vi "Passing Paramters Complex Struct.vi"(7 "y":i32, 9 "x":i32, 10 "numVertices":i32, 11 "name":u32) -> (3 "function return":i32)   [LabVIEW 2018, in "ParsingDataSampleDLL.lvlib"]
doc: "__declspec(dllexport) int PassingParamters_ComplexStruct (struct complexStructPolygon triangle);"
uses:
  ParsingDataSampleDLL.lvlib
  ni_reference_vs/Debug/ParsingDataSampleDLL.dll
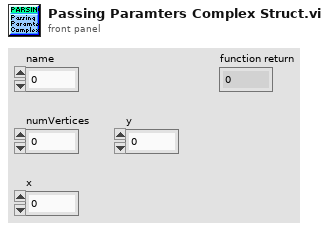
[diagram p1: front panel]
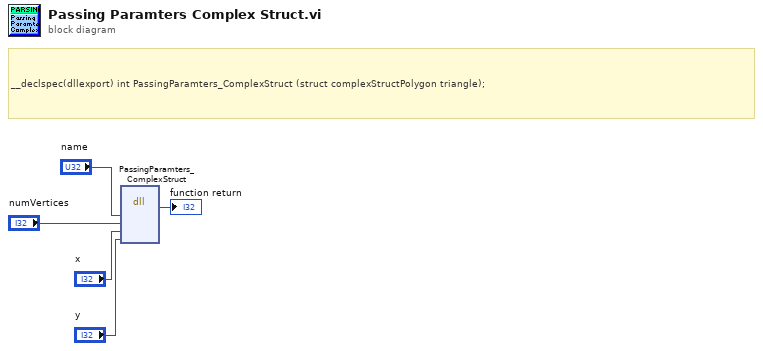
[diagram p0: block diagram]
diagram:
  # "__declspec(dllexport) int PassingParamters_ComplexStruct (struct complexStructPolygon triangle);"
  n1 = dll-call lib="C:/Users/celit/Documents/GitHub/Labview_Python_DLL_Call/ni_reference_vs/Debug/ParsingDataSampleDLL.*" fn="PassingParamters_ComplexStruct"("name"="name", "numVertices"="numVertices", "x"="x", "y"="y") -> (→"function return":i32)  [unwired: 7 in, 2 out]
